vi "1B Spoof Centripital Acceleration 2.vi"(6 "time elapsed since last iteration":dbl, 8 "Robot Velocity":T2, 9 "dHeading/dT in":T1 format="%05.1f", 10 "Robot\nHeading in":T1 format="%05.1f", 11 "Rudder Angle":T3) -> (1 "Robot\nHeading out":T1 format="%05.1f", 2 "dHeading":T3, 3 "dHeading/dT":T1 format="%05.1f")   [LabVIEW 2011]
uses:
  2-Think/2 Typedefs/rudder angle.ctl
  2-Think/2 Typedefs/heading.ctl
  2-Think/2 Typedefs/Velocity.ctl
  <vilib>/Analysis/coordinate.llb/Angle Units.ctl
  <vilib>/Analysis/coordinate.llb/Wrap Angle (scalar).vi
  <vilib>/Analysis/NI_AAL_Angle.lvlib
panel:
  out "Boolean":bool
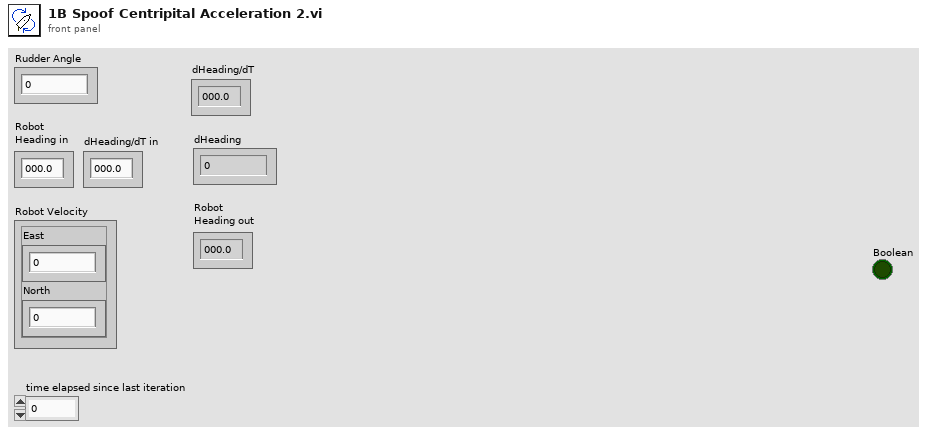
[diagram p1: front panel]
types:
  T1 = typedef "heading.ctl" = dbl
  T2 = typedef "Velocity.ctl" = cluster{"East":dbl, "North":dbl}
  T3 = typedef "rudder angle.ctl" = dbl
  T4 = typedef "NI_AAL_Angle.lvlib/Angle Units.ctl" = i32
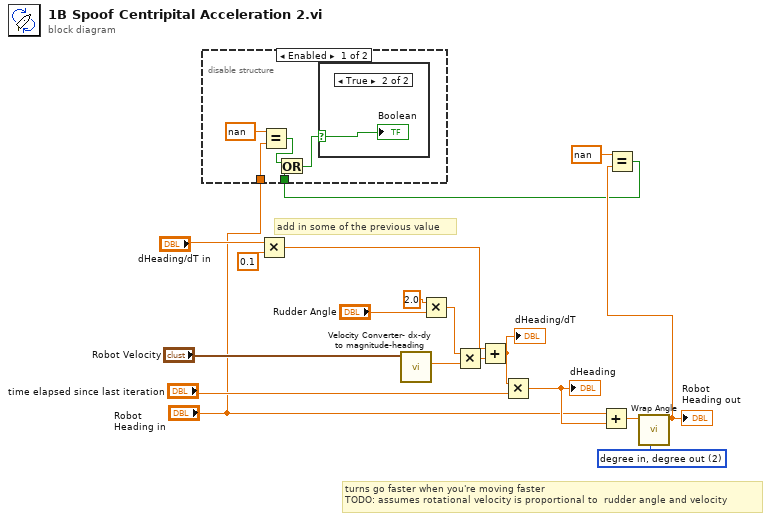
[diagram p0: block diagram]
diagram:
  w7 = T4 2 items=["radian in, radian out", "radian in, degree out", "degree in, degree out", "degree in, radian out"] ("angle units")
  # "add in some of the previous value"
  # "turns go faster when you're moving faster\nTODO: assumes rotational velocity is proportional to  rudder angle and velocity"
  n1 = Multiply(x="dHeading/dT in", y=T1 0.1) -> (x*y=w9:T1)
  n2 = call "Velocity Converter- dx-dy to magnitude-heading.vi"("Vector In"="Robot Velocity") -> ("Magnitude Out"=w15:dbl)  [unwired: 9 in, 1 out]
  n3 = Multiply(x=T3 2.0, y="Rudder Angle") -> (x*y=w6:T3)
  n4 = Multiply(x=w6, y=w15) -> (x*y=w13:T3)
  n5 = Add(x=w9, y=w13) -> (x+y=w10:T1)
  "dHeading/dT" <- w10
  n6 = Multiply(x=w10, y="time elapsed since last iteration") -> (x*y=w18:T1)
  "dHeading" <- w18
  n7 = Add(x="Robot\nHeading in", y=w18) -> (x+y=w8:T1)
  n8 = call-poly <vilib>:"Wrap Angle.vi"("angle units"=w7, "angle in"=w8) -> ("angle out"=w3:dbl)  [unwired: 8 in, 1 out]
  "Robot\nHeading out" <- w3
  n9 = Equal?(x=nan, y=w3) -> (x = y?=w1:bool)
  n10 = disable-structure shown="Enabled" {
    disable-tunnel: "Robot\nHeading in" -> [w22 _]
    disable-tunnel: w1 -> [w19 _]
    frame Enabled {
      n11 = Equal?(x=nan, y=w22) -> (x = y?=w21:bool)
      n12 = Or(x=w21, y=w19) -> (x .or. y?=w20:bool)
      n13 = case shown="True" w20 {
        selector: w20 -> [_ w24]
        frame False {
        }
        frame True {
          "Boolean" <- w24
        }
      }
    }
    frame Disabled {
    }
  }
